vi "brc_daq_start_DAQ.vi"(2 "rawValue":u8, 5 "error in (no error)":errorcluster, 6 "mHandle":i32) -> (19 "error out":errorcluster)   [LabVIEW 2019, in "BRC-DAQ x86.lvlib"]
uses:
  BRC-DAQ x86.lvlib
  DLL/brc_daq_sdk.dll
panel:
  out "return_value":i32
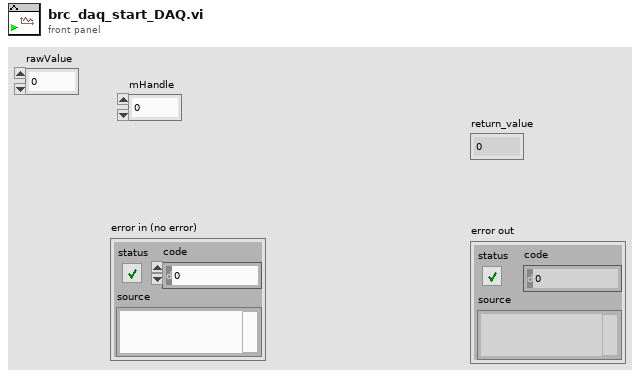
[diagram p1: front panel]
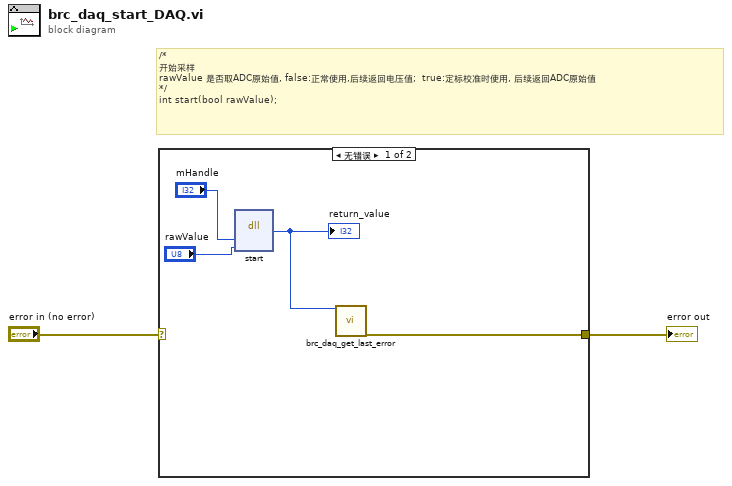
[diagram p0: block diagram]
diagram:
  # "/*\n开始采样\nrawValue 是否取ADC原始值, false:正常使用,后续返回电压值;  true:定标校准时使用, 后续返回ADC原始值\n*/\nint start(bool rawValue);"
  n1 = case shown="无错误" "error in (no error)" {
    selector: "error in (no error)" -> [_ w7]
    tunnel: [w5 w7] -> w2
    frame No Error {
      n2 = dll-call lib="E:/01 BRC project/04BRC-daq/04 git/test111/DLL/brc_daq_sdk.dll" fn="start"("mHandle"="mHandle", "rawValue"="rawValue") -> ("return type"=w6:i32)  [unwired: 5 in, 2 out]
      "return_value" <- w6
      n3 = call "brc_daq_get_last_error.vi"("return_value"=w6) -> ("error out"=w5:errorcluster)  [unwired: 18 in]
    }
    frame Error {
    }
  }
  "error out" <- w2
